vi "Modify_VIPB_Display_Information.vi"   [LabVIEW 2021]
uses:
  <vilib>/JDP Science/JSONtext/LVClass Serializer/JSONtext LVClass Serializer.lvclass
  <vilib>/Wiresmith Technology/G CLI/CLI Class/CLI.lvclass
  <vilib>/JKI/VIPM API/VIPM API_vipm_api.lvlib
  4199a0e4-84aa-42fd-b3f5-f9ce2ee7846d.vi
  <vilib>/JKI/VIPM API/command-line/support/Version Info Cluster_vipm_api.ctl
  <vilib>/JKI/VIPM API/command-line/support/VI Package Build Spec Data Cluster_vipm_api.ctl
types:
  T1 = enum32{"Invalid", "Standard", "Closed", "Hidden", "Minimized", "Maximized"}
  T2 = typedef "VIPM API_vipm_api.lvlib/VI Package Build Spec Data Cluster_vipm_api.ctl" = cluster{"Package Version":T3, "Product Name":string, "Company Name":string, "Author Name (Person or Company)":string, "Product Homepage (URL)":string, "Legal Copyright":string, "License Agreement Name":string, "Product Description Summary":string, "Product Description":string, "Release Notes - Change Log":string}
  T3 = typedef "VIPM API_vipm_api.lvlib/Version Info Cluster_vipm_api.ctl" = cluster{"major":u32, "minor":u32, "patch":u32, "build":u32}
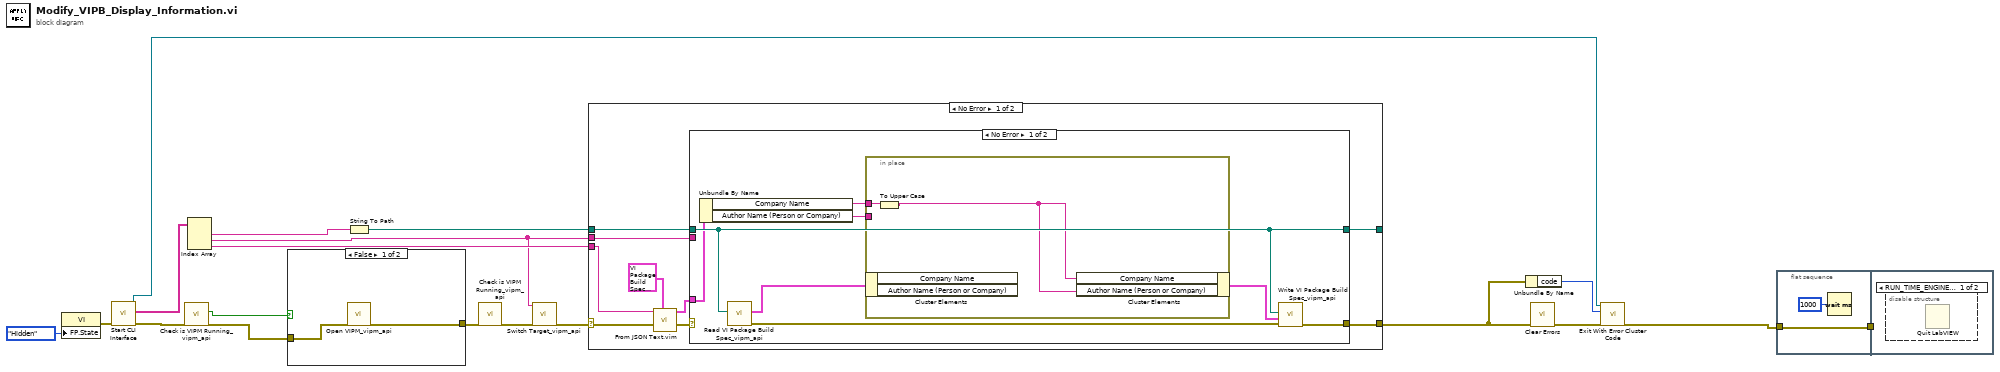
[diagram p0: block diagram]
diagram:
  n1 = property class="VI"("FP.State"=T1."Hidden" ("Front Panel Window:State")) -> (error out=w18:errorcluster)  [unwired: 2 in, 1 out]
  n2 = call <vilib>:"Start CLI Interface.vi"("error in (no error)"=w18) -> ("error out"=w10:errorcluster, "Custom Parameters"=w15:string[], "CLI out"=w17:refnum<class "CLI.lvclass">)  [unwired: 7 in, 1 out]
  n3 = call <vilib>:"Check is VIPM Running_vipm_api.vi"("error in (no error)"=w10) -> ("error out"=w16:errorcluster, "is Running"=w7:bool)  [unwired: 9 in]
  n4 = Index Array(array=w15) -> (element #1=w11:string, element #2=w2:string, element #3=w9:string)  [unwired: 3 in]
  n5 = case shown="False" w7 {
    tunnel: w16 -> [w21 w22]
    tunnel: [w20 w22] -> w6
    frame False {
      n6 = call <vilib>:"Open VIPM_vipm_api.vi"("error in (no error)"=w21) -> ("error out"=w20:errorcluster)  [unwired: 10 in]
    }
    frame True {
    }
  }
  n7 = String To Path(string=w11) -> (path=w8:path)
  n8 = call <vilib>:"Check is VIPM Running_vipm_api.vi"("error in (no error)"=w6) -> ("error out"=w4:errorcluster)  [unwired: 9 in, 1 out]
  n9 = call <vilib>:"Switch Target_vipm_api.vi"("error in (no error)"=w4, "LabVIEW Version"=w2) -> ("error out"=w3:errorcluster)  [unwired: 9 in]
  n10 = case shown="No Error" w3 {
    selector: w3 -> [w31 w44]
    tunnel: w9 -> [w30 _]
    tunnel: w8 -> [w25 w43]
    tunnel: w2 -> [w24 _]
    tunnel: [w27 w44] -> w1
    tunnel: [w23 w43] -> _
    frame No Error {
      n11 = call "From JSON Text.vim"("Data Type and Default Value"=T2 {"Package Version"={"major"=0, "minor"=0, "patch"=0, "build"=0}, "Product Name"="", "Company Name"="", "Author Name (Person or Company)"="", "Product Homepage (URL)"="", "Legal Copyright"="", "License Agreement Name"="", "Product Description Summary"="", "Product Description"="", "Release Notes - Change Log"=""} ("VI Package Build Spec Data"), "error in (no error)"=w31, "JSON"=w30) -> ("error out"=w29:errorcluster, "Data out"=w26:T2)  [unwired: 7 in]
      n12 = case shown="No Error" w29 {
        tunnel: [w39 _] -> w27
        tunnel: w26 -> [w35 _]
        tunnel: w25 -> [w38 w42]
        tunnel: w24 -> [_ _]
        tunnel: [w38 w42] -> w23
        frame No Error {
          n13 = Unbundle By Name(w35) -> ("Company Name"=w34:string, "Author Name (Person or Company)"=w33:string)
          n14 = call <vilib>:"Read VI Package Build Spec_vipm_api.vi"("Path to VIPB File"=w38) -> ("error out"=w37:errorcluster, "VI Package Build Spec Data"=w36:T2)  [unwired: 9 in]
          n15 = in-place {
            in-place-border: w34 -> [w41]
            in-place-border: w33 -> [_]
            n16 = in-place-cluster #1(w36) -> ()  [unwired: 2 out]
            n17 = To Upper Case(1:w41) -> (0:w40:string)
            n18 = in-place-cluster #1("Company Name"=w40, "Author Name (Person or Company)"=w40) -> (w32:T2)
          }
          n19 = call <vilib>:"Write VI Package Build Spec_vipm_api.vi"("error in (no error)"=w37, "VI Package Build Spec Data"=w32, "Path to VIPB File"=w38) -> ("error out"=w39:errorcluster)  [unwired: 8 in]
        }
        frame Error {
        }
      }
    }
    frame Error {
    }
  }
  n20 = Unbundle By Name(w1) -> ("code"=w12:i32)
  n21 = call <vilib>:"Clear Errors.vi"("error in (no error)"=w1) -> ("error out"=w5:errorcluster)  [unwired: 5 in, 1 out]
  n22 = call <vilib>:"Exit With Error Cluster Code.vi"("error in (no error)"=w5, "No Error Code (0)"=w12, "CLI in"=w17) -> ("error out"=w13:errorcluster)  [unwired: 8 in]
  n23 = flat-sequence {
    tunnel: w13 -> [w46]
    tunnel: [w46] -> w14
    tunnel: w14 -> [_]
    frame #0 {
      n24 = Wait (ms)(milliseconds to wait=u32 1000) -> ()  [unwired: 1 out]
    }
    frame #1 {
      n25 = disable-structure shown="RUN_TIME_ENGINE==True" {
        frame condition #0 {
          n26 = Quit LabVIEW() -> ()  [unwired: 1 in]
        }
        frame condition #1 (active) {
        }
      }
    }
  }
